vi "Disconnect.vi"(8 "error in (no error)":errorcluster, 10 "Disconnection list in":string, 11 "SLSC Switch Consumer in":refnum<class "SLSC Switch Consumer.lvclass">) -> (0 "error out":errorcluster, 3 "SLSC Switch Consumer out":refnum<class "SLSC Switch Consumer.lvclass">)   [LabVIEW 2020, in "SLSC Switch Messaging.lvlib" / "SLSC Switch Consumer.lvclass"]
uses:
  SLSC Switch Consumer.lvclass
  SLSC Switch Consumer.lvclass/SLSC Switch Consumer.ctl
  <vilib>/SLSC_Switch/Disconnect Channels (Multiple).vi
  <vilib>/SLSC_Switch/SLSC Switch.lvlib
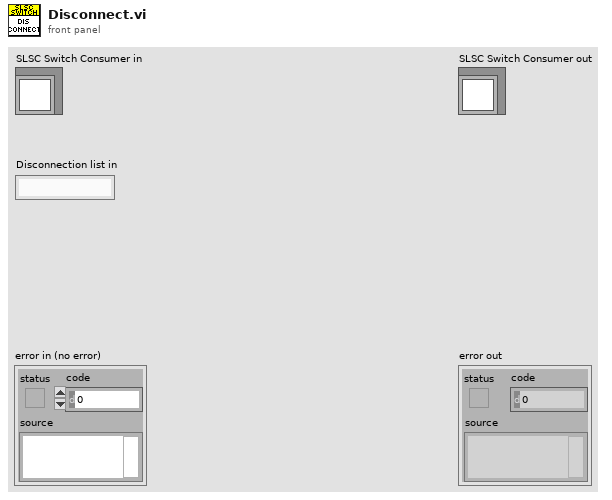
[diagram p1: front panel]
types:
  T1 = typedef "nislscslSession.ctl" = refnum<k20>
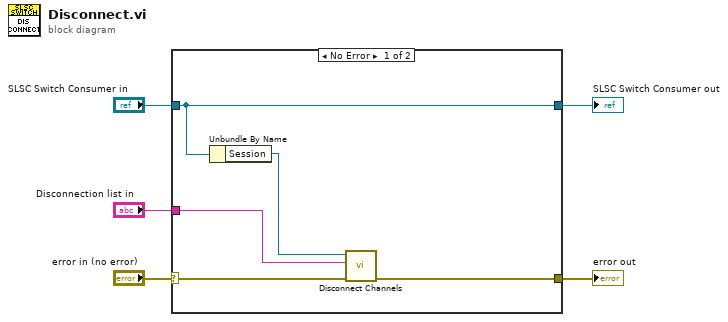
[diagram p0: block diagram]
diagram:
  n1 = case shown="No Error" "error in (no error)" {
    selector: "error in (no error)" -> [w7 w12]
    tunnel: [w6 w12] -> w3
    tunnel: [w10 w11] -> w1
    tunnel: "SLSC Switch Consumer in" -> [w10 w11]
    tunnel: "Disconnection list in" -> [w9 _]
    frame No Error {
      n2 = Unbundle By Name(w10) -> ("Session"=w8:T1)
      n3 = call-poly <vilib>:"Disconnect Channels.vi"("error in (no error)"=w7, "disconnection list"=w9, "session in"=w8) -> ("error out"=w6:errorcluster)  [unwired: 7 in, 1 out]
    }
    frame Error {
    }
  }
  "error out" <- w3
  "SLSC Switch Consumer out" <- w1
